vi "Write Radio Buttons.vi"(8 "error in":errorcluster, 10 "Value":string[](array[string]), 11 "Radio Buttons Reference in":refnum<vi>) -> (0 "error out":errorcluster, 3 "Radio Buttons Reference out":refnum<vi>)   [LabVIEW 2020, in "G-Unicode.lvlib"]
uses:
  G-Unicode.lvlib
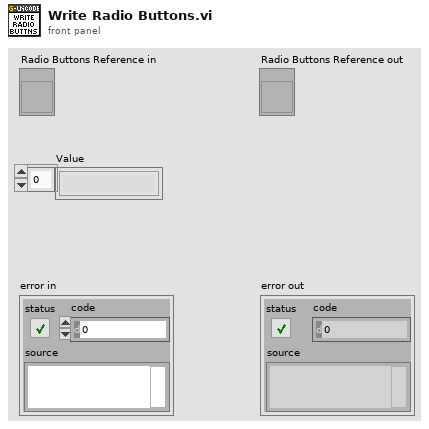
[diagram p1: front panel]
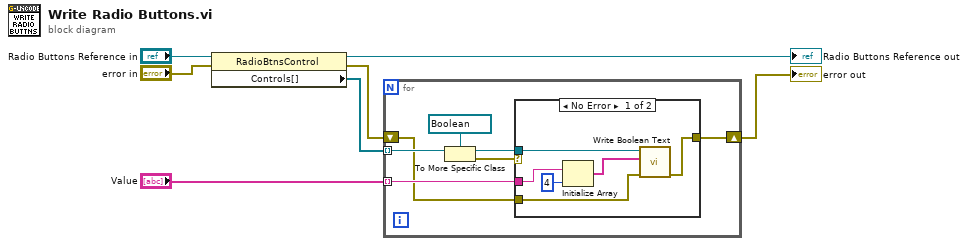
[diagram p0: block diagram]
diagram:
  n1 = property class="RadioBtnsControl"(reference="Radio Buttons Reference in", error in="error in") -> (reference out=→"Radio Buttons Reference out":refnum<vi>, error out=w3:errorcluster, "Controls[]"=w6:refnum<vi>[])
  n2 = for {
    tunnel: w6 -> [w14] mode=indexing
    tunnel: "Value" -> [w10] mode=indexing
    shift-right: [w8] -> w2
    shift-left: w3 -> [w9]
    n3 = To More Specific Class(target class=refnum<vi> refnum ("Boolean Reference in"), reference=w14) -> (specific class reference=w11:refnum<vi>, error out=w12:errorcluster)  [unwired: 1 in]
    n4 = case shown="No Error" w12 {
      tunnel: w11 -> [w20 _]
      tunnel: w10 -> [w19 _]
      tunnel: w9 -> [w16 w21]
      tunnel: [w15 w21] -> w8
      frame No Error {
        n5 = Initialize Array(w19, 4 ("dimension size")) -> (w18:string[])
        n6 = call "Write Boolean Text.vi"("error in"=w16, "Value"=w18, "Boolean Reference in"=w20) -> ("error out"=w15:errorcluster)  [unwired: 7 in, 1 out]
      }
      frame Error {
      }
    }
  }
  "error out" <- w2
